vi "Write ENG.vi"(8 "error in (no error)":errorcluster, 10 "ENG":bool, 11 "Mensajes Actor in":refnum<class "Mensajes Actor.lvclass">) -> (0 "error out":errorcluster, 3 "Mensajes Actor out":refnum<class "Mensajes Actor.lvclass">)   [LabVIEW 2019, in "Mensajes Actor.lvlib" / "Mensajes Actor.lvclass"]
uses:
  Mensajes Actor.lvclass
  Mensajes Actor.lvclass/Mensajes Actor.ctl
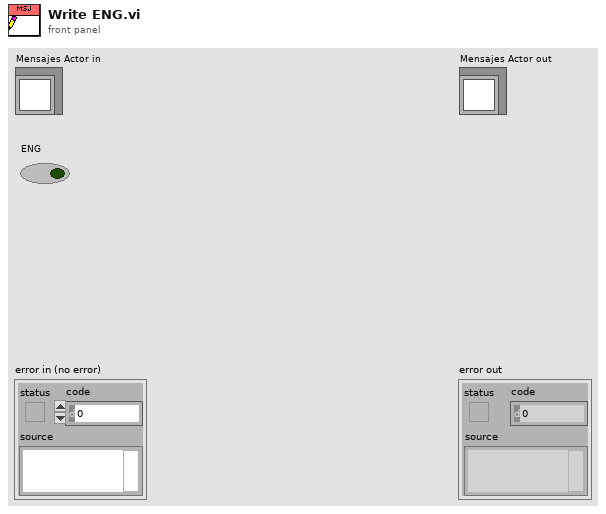
[diagram p1: front panel]
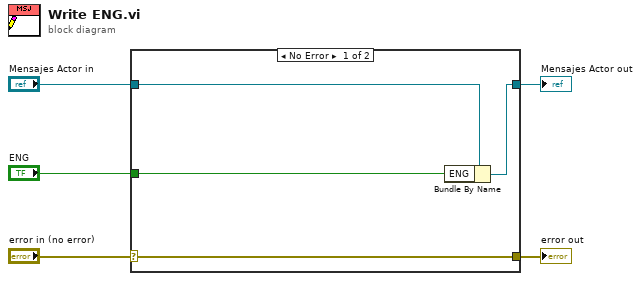
[diagram p0: block diagram]
diagram:
  n1 = case shown="No Error" "error in (no error)" {
    selector: "error in (no error)" -> [w9 w10]
    tunnel: [w9 w10] -> w4
    tunnel: [w7 w11] -> w2
    tunnel: "Mensajes Actor in" -> [w8 w11]
    tunnel: "ENG" -> [w6 _]
    frame No Error {
      n2 = Bundle By Name(cluster=w8, "ENG"=w6) -> (w7:refnum<class "Mensajes Actor.lvclass">)
    }
    frame Error {
    }
  }
  "error out" <- w4
  "Mensajes Actor out" <- w2
